vi "Launch.vi"(7 "Common Config":T1={"Launch Timeout [ms]"=-1, "Wait For Launch Completed"=FALSE, "Front Panel State"=enum."Standard", "Close FP On Shutdown"=TRUE, "Response Channel"=refnum, "Sub Panel"=refnum}, 8 "error in (no error)":errorcluster, 10 "Maximum Number Of Errors":i32, 11 "Definitions":path) -> (0 "error out":errorcluster, 3 "Launch Time":timestamp)   [LabVIEW 2015, in "Alarm Handler Actor.lvclass"]
doc: "<b>Response</b> channel is used by this actor to return infomation back to the parent. Typically this input is the Request channel of the parent actor."
uses:
  Alarm Handler Actor.lvclass
  Re-use Libraries/Minimal Actor Framework/Actors/Base Actor/Actor/Common Config.ctl
  Re-use Libraries/Minimal Actor Framework/Messaging/Messenger/Messenger.lvclass
  Re-use Libraries/Minimal Actor Framework/Actors/Base Actor/Actor/Front Panel State.ctl
  API/Alarm Handler Actor API.lvclass
  Alarm Handler Actor.lvclass/Alarm Handler Actor.ctl
  Globals.vi
  Re-use Libraries/Minimal Actor Framework/Actors/Base Actor/API/Actor API.lvclass
  Re-use Libraries/Minimal Actor Framework/Actors/Base Actor/Actor/Actor.lvclass
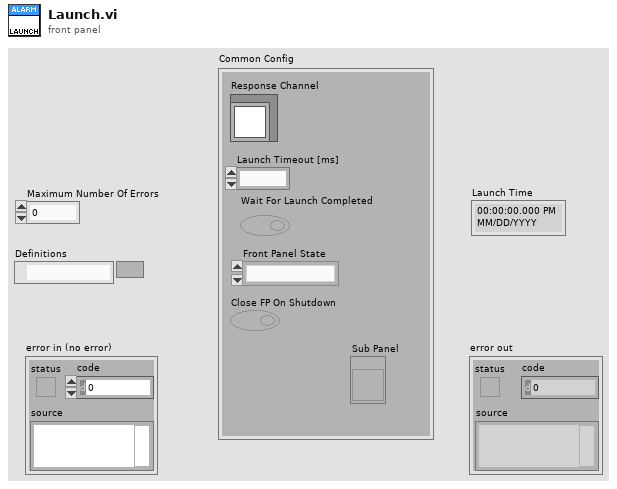
[diagram p1: front panel]
types:
  T1 = typedef "Actor.lvclass/Common Config.ctl" = cluster{"Launch Timeout [ms]":i32, "Wait For Launch Completed":bool, "Front Panel State":T2, "Close FP On Shutdown":bool, "Response Channel":refnum<class "Messenger.lvclass">, "Sub Panel":refnum<vi>}
  T2 = typedef "Actor.lvclass/Front Panel State.ctl" = enum32{"Invalid", "Standard", "Closed", "Hidden", "Minimized", "Maximized"}
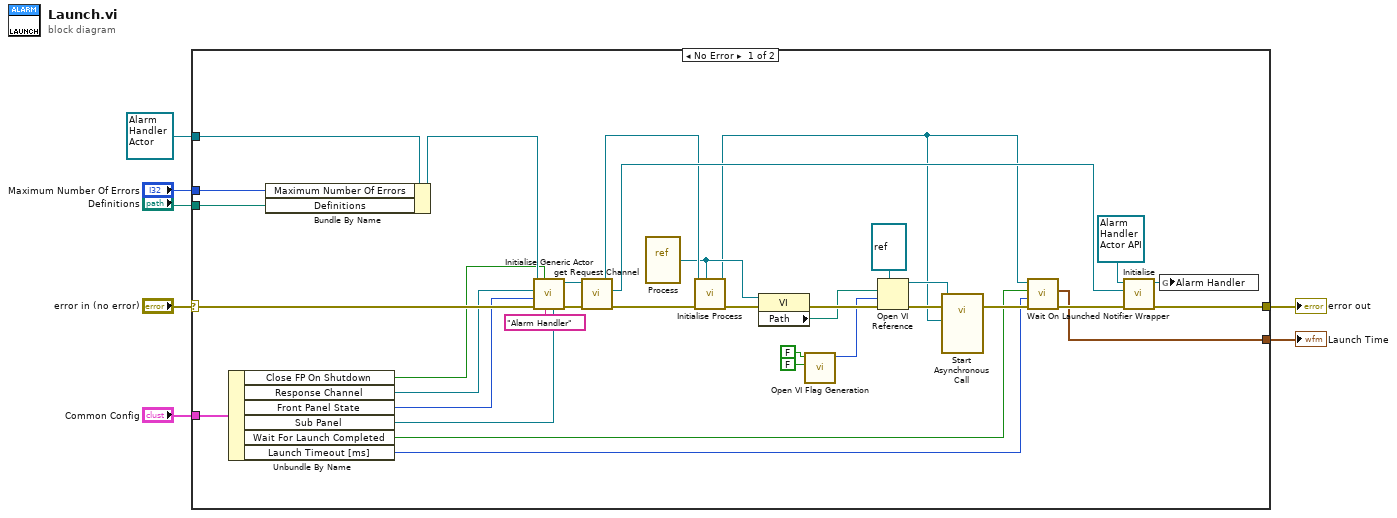
[diagram p0: block diagram]
diagram:
  n1 = case shown="No Error" "error in (no error)" {
    selector: "error in (no error)" -> [w38 w42]
    tunnel: [w37 w42] -> w7
    tunnel: refnum<class "Alarm Handler Actor.lvclass"> refnum ("Worker Test 1.lvclass") -> [w36 _]
    tunnel: "Maximum Number Of Errors" -> [w34 _]
    tunnel: [w32 _] -> w3
    tunnel: "Definitions" -> [w15 _]
    tunnel: "Common Config" -> [w14 _]
    frame No Error {
      n2 = Unbundle By Name(w14) -> ("Close FP On Shutdown"=w13:bool, "Response Channel"=w12:refnum<class "Messenger.lvclass">, "Front Panel State"=w11:T2, "Sub Panel"=w10:refnum<vi>, "Wait For Launch Completed"=w9:bool, "Launch Timeout [ms]"=w8:i32)
      n3 = Bundle By Name(cluster=w36, "Maximum Number Of Errors"=w34, "Definitions"=w15) -> (w35:refnum<class "Alarm Handler Actor.lvclass">)
      n4 = call-dynamic "Initialise Generic Actor.vi"("Sub Panel"=w10, "Name"="Alarm Handler", "Close FP On Shutdown (T)"=w13, "Front Panel State"=w11, "Response Channel"=w12, "Actor in"=w35) -> ("Actor out"=w39:refnum<class "Alarm Handler Actor.lvclass">)  [unwired: 4 in, 1 out]
      n5 = call "get Request Channel.vi"("error in (no error)"=w38, "Actor in"=w39) -> ("error out"=w21:errorcluster, "Request Channel"=w41:refnum<class "Messenger.lvclass">, "Actor out"=w19:refnum<class "Alarm Handler Actor.lvclass">)  [unwired: 7 in]
      n6 = vi-ref "Process.vi"() -> (w18:refnum<vi>)
      n7 = call-dynamic "Initialise Process.vi"("Process"=w18, "error in (no error)"=w21, "Actor in"=w19) -> ("error out"=w30:errorcluster, "Actor out"=w17:refnum<class "Alarm Handler Actor.lvclass">)  [unwired: 7 in]
      n8 = property class="VI"(reference=w18, error in=w30) -> (error out=w29:errorcluster, "Path"=w22:path)  [unwired: 1 out]
      n9 = call "Open VI Flag Generation.vi"("Call And Collect (F)"=FALSE, "Re-entrant (F)"=FALSE) -> ("Flags"=w28:i32)  [unwired: 9 in]
      n10 = Open VI Reference(type specifier VI Refnum (for type only)=refnum<vi> refnum, vi path=w22, options=w28, error in (no error)=w29) -> (vi reference=w24:refnum<vi>, error out=w23:errorcluster)  [unwired: 2 in]
      n11 = call-by-ref "Start Asynchronous Call"(reference=w24, error in=w23, "Actor"=w17) -> (error out=w20:errorcluster)  [unwired: 11 in, 1 out]
      n12 = call-dynamic "Wait On Launched Notifier Wrapper.vi"("error in (no error)"=w20, "Launch Timeout [ms]"=w8, "Wait For Launch Completed"=w9, "Actor in"=w17) -> ("error out"=w33:errorcluster, "Launch Time"=w32:timestamp)  [unwired: 5 in, 1 out]
      n13 = call "Initialise.vi"("error in (no error)"=w33, "Request Channel"=w41, "Actor API in"=refnum<class "Alarm Handler Actor API.lvclass"> refnum ("Actor API")) -> ("error out"=w37:errorcluster, "Actor API out"=w16:refnum<class "Alarm Handler Actor API.lvclass">)  [unwired: 7 in]
      n14 = global write "Globals.vi" "Alarm Handler"(w16) -> ()
    }
    frame Error {
    }
  }
  "error out" <- w7
  "Launch Time" <- w3
